vi "telemetry.vi"   [LabVIEW 2015]
uses:
  <vilib>/rvi/Emulation/niFpgaEmulationIsFPGAContextNoSignature.vi
  <vilib>/rvi/FIFO/Fifo_Resource/nirvififoEmulationSetSize.vi
  <vilib>/rvi/DataTransferAndStorage/Container/Common/niFpgaContainerGetUniqueNameForEmu.vi
  <vilib>/rvi/FIFO/Fifo_Resource/nirviFifoEmulationQueueMgr.vi
  <instcachedir>/0/nirviFifoEmulationQueueMgr_E5CAEC123FF24DC58D834DCA3CDAA9B5.lvgen/nirviFifoEmulationQueueMgr_E5CAEC123FF24DC58D834DCA3CDAA9B5_008.vi
  <vilib>/rvi/Emulation/niFpgaProcessEmulError.vi
  <vilib>/rvi/DataTransferAndStorage/Container/XNode/niFpgaContainer.xnode
  <vilib>/rvi/FIFO/Fifo_Resource/nirvififoEmulationClear.vi
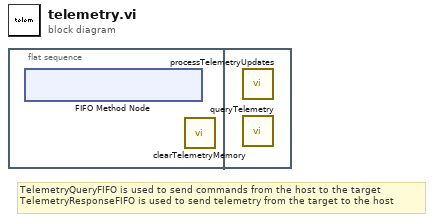
[diagram p0: block diagram]
diagram:
  # "TelemetryQueryFIFO is used to send commands from the host to the target\nTelemetryResponseFIFO is used to send telemetry from the target to the host"
  n1 = flat-sequence {
    frame #0 {
      n2 = xnode ("FIFO Method Node")() -> ()  [unwired: 1 in, 1 out]
      n3 = call "clearTelemetryMemory.vi"() -> ()  [unwired: 12 in]
    }
    frame #1 {
      n4 = call "processTelemetryUpdates.vi"() -> ()  [unwired: 12 in]
      n5 = call "queryTelemetry.vi"() -> ()  [unwired: 12 in]
    }
  }
